vi "FTW-Regex-ForceLiteral.vi"(0 "Input":string, 1 "Force Literal Match?":bool=TRUE) -> (2 "Output":string)   [LabVIEW 2013]
panel:
  # "Inputs"
  # "Outputs"
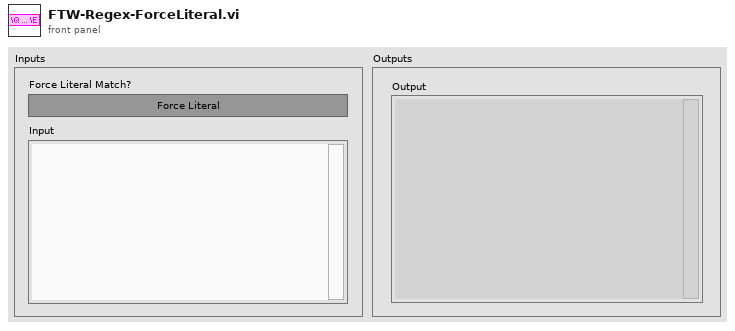
[diagram p1: front panel]
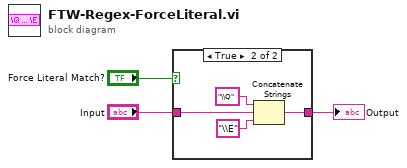
[diagram p0: block diagram]
diagram:
  n1 = case shown="True" "Force Literal Match?" {
    tunnel: "Input" -> [w4 w6]
    tunnel: [w4 w5] -> w2
    frame False {
    }
    frame True {
      n2 = Concatenate Strings("\\Q", w6, "\\E") -> (w5:string)
    }
  }
  "Output" <- w2
